vi "AutoDrive.vi"(8 "Drive Time":u32, 9 "Drive Speed":dbl, 10 "Wait before drive":u32, 11 "Motor Name":string="RobotDrive") -> ()   [LabVIEW 2017]
uses:
  <vilib>/Rock Robotics/WPI/Utilities/WPI_GetSetVariantRefNum.vi
  <vilib>/Rock Robotics/WPI/RobotDrive/WPI_RobotDriveArcadeDrive_Standard(NoSaturation).vi
panel:
  # "Sample autonomous program to drive forward for set amount of time"
  # "Click Window->Show block diagram to view the rest of the code"
  # "This program waits for entered time, drives for time @ speed, then stops"
  # "WAIT"
  # "DRIVE"
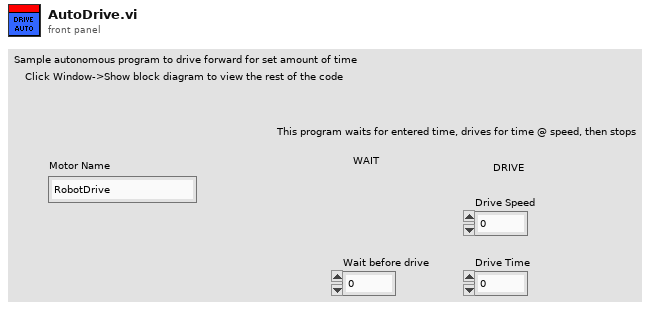
[diagram p1: front panel]
types:
  T1 = typedef "WPI_RobotDriveDevRef.ctl" = cluster{"DevStatus":errorcluster, "Motors[]":T2[], "Square Inputs":bool, "Max Output":dbl}
  T2 = typedef "WPI_MotorControlDeviceRef.ctl" = cluster{"DeviceStatus":errorcluster, "Type":T3, "PWM":cluster{"PWM Channel":T4, "DeadBand":T5}, "CAN":cluster{"Device Number":u8, "SetOutput VI Ref":variant, "GetOutput VI Ref":variant, "Enable VI Ref":variant, "Disable VI Ref":variant, "Data":variant}, "Invert":bool, "DIO PWM":cluster{"PWM \"Enable\" Channel":T4, "DIOChannel":T6, "PWM Rate":dbl}}
  T3 = typedef "WPI_MotorControlType.ctl" = enum16{"PWM", "CAN", "DIO PWM"}
  T4 = typedef "FPGA_DIOPWMChannel.ctl" = enum8{"PWM 0", "PWM 1", "PWM 2", "PWM 3", "PWM 4", "PWM 5", "PWM 6", "PWM 7", "PWM 8", "PWM 9", "PWM MXP 0", "PWM MXP 1", "PWM MXP 2", "PWM MXP 3", "PWM MXP 4", "PWM MXP 5", "PWM MXP 6", "PWM MXP 7", "PWM MXP 8", "PWM MXP 9", "Invalid"}
  T5 = typedef "WPI_PWMDeadband.ctl" = cluster{"Name":string, "maxPositivePwm":i32, "minPositivePwm":i32, "centerPwm":i32, "maxNegativePwm":i32, "minNegativePwm":i32, "angularRange":u16}
  T6 = typedef "FPGA_DIOChannel.ctl" = enum8{"DIO 0", "DIO 1", "DIO 2", "DIO 3", "DIO 4", "DIO 5", "DIO 6", "DIO 7", "DIO 8", "DIO 9", "DIO MXP 0", "DIO MXP 1", "DIO MXP 2", "DIO MXP 3", "DIO MXP 4", "DIO MXP 5", "DIO MXP 6", "DIO MXP 7", "DIO MXP 8", "DIO MXP 9", "DIO MXP 10", "DIO MXP 11", "DIO MXP 12", "DIO MXP 13", "DIO MXP 14", "DIO MXP 15", "SPI Port CS1", "SPI Port CS2", "SPI Port CS3", "SPI Port MISO", "SPI Port MOSI", "Invalid"}
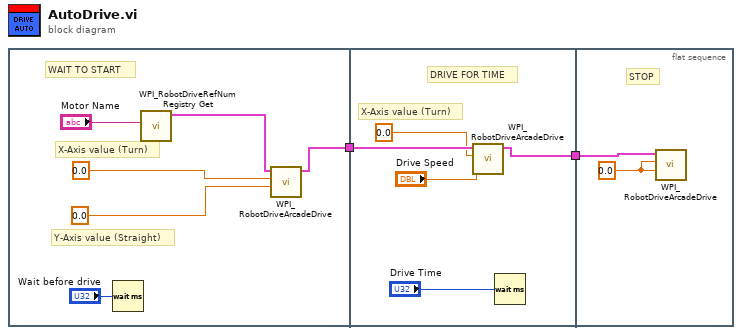
[diagram p0: block diagram]
diagram:
  n1 = flat-sequence {
    tunnel: [w5] -> w2
    tunnel: w2 -> [w13]
    tunnel: [w9] -> w1
    tunnel: w1 -> [w15]
    frame #0 {
      # "WAIT TO START"
      # "Y-Axis value (Straight)"
      # "X-Axis value (Turn)"
      n2 = Wait (ms)(milliseconds to wait="Wait before drive") -> ()  [unwired: 1 out]
      n3 = call <vilib>:"WPI_RobotDriveRefNum Registry Get.vi"("refnum name"="Motor Name") -> ("RobotDriveDevRef"=w8:T1)  [unwired: 9 in, 1 out]
      n4 = call-poly <vilib>:"WPI_RobotDriveArcadeDrive.vi"("Y axis value"=0.0, "X axis value"=0.0, "RobotDriveDevRef"=w8) -> ("RobotDriveDevRef"=w5:T1)  [unwired: 6 in, 2 out]
    }
    frame #1 {
      # "DRIVE FOR TIME"
      # "X-Axis value (Turn)"
      n5 = call-poly <vilib>:"WPI_RobotDriveArcadeDrive.vi"("Y axis value"="Drive Speed", "X axis value"=0.0, "RobotDriveDevRef"=w13) -> ("RobotDriveDevRef"=w9:T1)  [unwired: 6 in, 2 out]
      n6 = Wait (ms)(milliseconds to wait="Drive Time") -> ()  [unwired: 1 out]
    }
    frame #2 {
      w14 = 0.0 ("Y axis value")
      # "STOP"
      n7 = call-poly <vilib>:"WPI_RobotDriveArcadeDrive.vi"("Y axis value"=w14, "X axis value"=w14, "RobotDriveDevRef"=w15) -> ()  [unwired: 6 in, 3 out]
    }
  }
